vi "Capture2DAnd3D.vi"(7 "error in (no error)":errorcluster, 8 "Camera Reference in":refnum<k24>) -> (0 "TexturedPointCloud Reference out":refnum<k24>, 1 "Frame2DAnd3D Reference out":refnum<k24>, 2 "UntexturedPointCloud Reference out":refnum<k24>, 3 "DepthMap Reference out":refnum<k24>, 4 "error out":errorcluster, 5 "Color2DImage Reference out":refnum<k24>, 6 "Camera Reference out":refnum<k24>)   [LabVIEW 2023]
uses:
  C:/Users/mech-mind/Downloads/LabView/MechEyeApiNet.dll
  MechEyeApiNet.dll
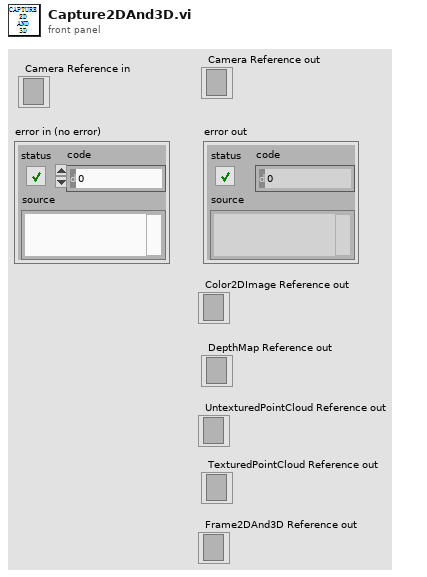
[diagram p1: front panel]
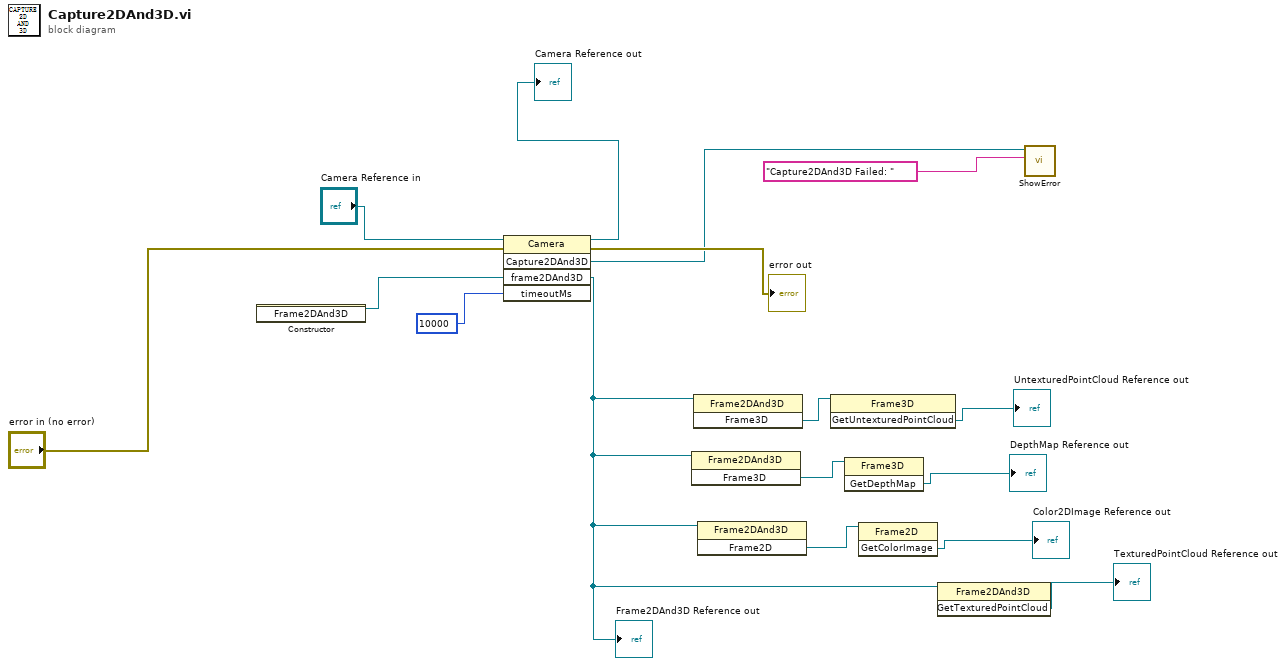
[diagram p0: block diagram]
diagram:
  n1 = constructor class="Frame2DAnd3D"() -> (reference out=w14:refnum<k24>)  [unwired: 3 in, 2 out]
  n2 = invoke class="Camera" method="Capture2DAnd3D"(reference="Camera Reference in", error in="error in (no error)", "frame2DAnd3D"=w14, "timeoutMs"=10000) -> (reference out=→"Camera Reference out":refnum<k24>, error out=→"error out":errorcluster, "Capture2DAnd3D"=w10:refnum<k24>, "frame2DAnd3D"=w11:refnum<k24>)  [unwired: 1 in, 1 out]
  "Frame2DAnd3D Reference out" <- w11
  n3 = invoke class="Frame2DAnd3D" method="Frame3D"(reference=w11) -> ("Frame3D"=w4:refnum<k24>)  [unwired: 2 in, 2 out]
  n4 = invoke class="Frame2DAnd3D" method="Frame3D"(reference=w11) -> ("Frame3D"=w6:refnum<k24>)  [unwired: 2 in, 2 out]
  n5 = invoke class="Frame2DAnd3D" method="Frame2D"(reference=w11) -> ("Frame2D"=w2:refnum<k24>)  [unwired: 2 in, 2 out]
  n6 = invoke class="Frame3D" method="GetUntexturedPointCloud"(reference=w6) -> ("GetUntexturedPointCloud"=→"UntexturedPointCloud Reference out":refnum<k24>)  [unwired: 2 in, 2 out]
  n7 = invoke class="Frame3D" method="GetDepthMap"(reference=w4) -> ("GetDepthMap"=→"DepthMap Reference out":refnum<k24>)  [unwired: 2 in, 2 out]
  n8 = invoke class="Frame2D" method="GetColorImage"(reference=w2) -> ("GetColorImage"=→"Color2DImage Reference out":refnum<k24>)  [unwired: 2 in, 2 out]
  n9 = invoke class="Frame2DAnd3D" method="GetTexturedPointCloud"(reference=w11) -> ("GetTexturedPointCloud"=→"TexturedPointCloud Reference out":refnum<k24>)  [unwired: 2 in, 2 out]
  n10 = call "ShowError.vi"("String"="Capture2DAnd3D Failed: ", "ErrorStatus Refnum in"=w10) -> ()  [unwired: 10 in]
